vi "Execute.vi"(8 "error in (no error)":errorcluster, 10 "Context in":refnum<class "Context.lvclass">, 11 "Stop Search For Zero in":refnum<class "Stop Search For Zero.lvclass">) -> (0 "error out":errorcluster, 2 "Context out":refnum<class "Context.lvclass">, 3 "Stop Search For Zero out":refnum<class "Stop Search For Zero.lvclass">)   [LabVIEW 2016, in "Stop Search For Zero.lvclass"]
uses:
  Stop Search For Zero.lvclass
  Context/Context.lvclass
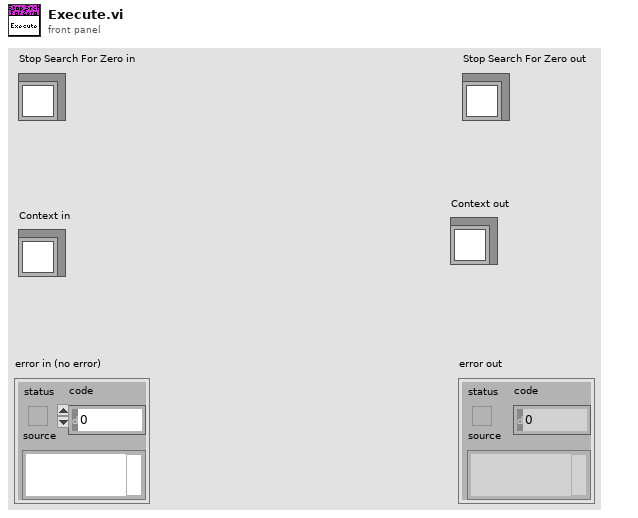
[diagram p1: front panel]
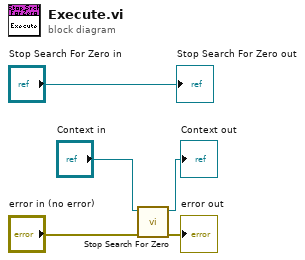
[diagram p0: block diagram]
diagram:
  n1 = call "Stop Search For Zero.vi"("error in (no error)"="error in (no error)", "Context in"="Context in") -> ("error out"=→"error out":errorcluster, "Context out"=→"Context out":refnum<class "Context.lvclass">)  [unwired: 8 in]
  "Stop Search For Zero out" <- "Stop Search For Zero in"
